vi "Read Stamps.vi"(8 "error in (no error)":errorcluster, 11 "WorkTable Class in":refnum<class "WorkTable Class.lvclass">) -> (0 "error out":errorcluster, 2 "Stamps":T1, 3 "WorkTable Class out":refnum<class "WorkTable Class.lvclass">)   [LabVIEW 2011, in "WorkTable Class.lvclass"]
uses:
  WorkTable Class.lvclass
  Vec3d Class/Vec3d Class.lvclass
  WorkTable Class.lvclass/WorkTable Class.ctl
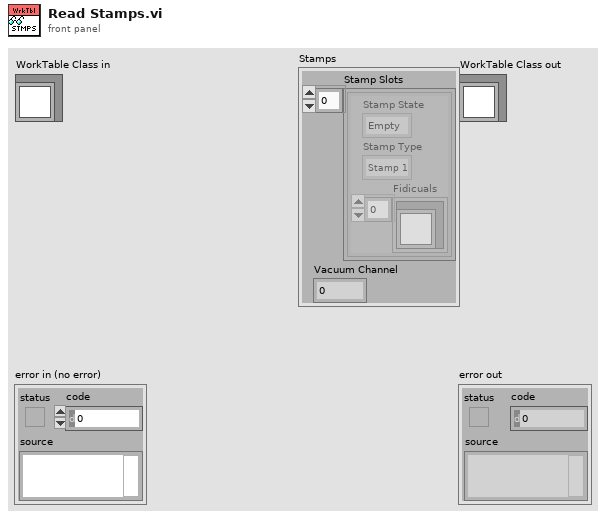
[diagram p1: front panel]
types:
  T1 = cluster{"Stamp Slots":cluster{"Stamp State":enum16{"Empty", "Populated", "Used"}, "Stamp Type":enum16{"Stamp 1", "Stamp 2", "Stamp 3", "Stamp 4"}, "Fidicuals":refnum<class "Vec3d Class.lvclass">[]}[], "Vacuum Channel":u8}
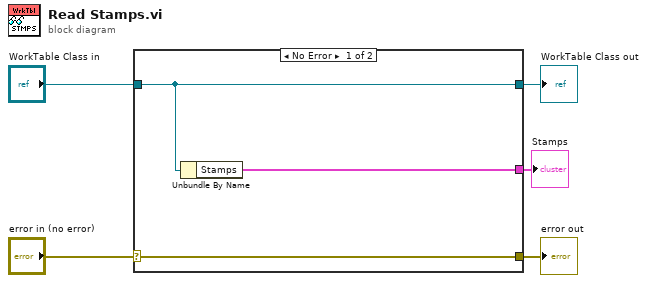
[diagram p0: block diagram]
diagram:
  n1 = case shown="No Error" "error in (no error)" {
    selector: "error in (no error)" -> [w8 w9]
    tunnel: [w8 w9] -> w4
    tunnel: [w7 w10] -> w2
    tunnel: "WorkTable Class in" -> [w7 w10]
    tunnel: [w6 _] -> w1
    frame No Error {
      n2 = Unbundle By Name(w7) -> ("Stamps"=w6:T1)
    }
    frame Error {
    }
  }
  "error out" <- w4
  "WorkTable Class out" <- w2
  "Stamps" <- w1
